vi "SendCTREPCMProtocol.vi"(7 "Send":bool, 9 "Initialize":bool, 10 "Previous":T1={"type"="CTREPCM", "device"="", "name"="", "data"={"<init"=FALSE, ">on"=FALSE, "<closed_loop"=FALSE, ">pressure_switch"=FALSE, ">current"=0.0}}, 11 "Current":T1={"type"="CTREPCM", "device"="", "name"="", "data"={"<init"=FALSE, ">on"=FALSE, "<closed_loop"=FALSE, ">pressure_switch"=FALSE, ">current"=0.0}}) -> ()   [LabVIEW 2019]
uses:
  CTREPCM Data proto.ctl
  CTREPCM proto.ctl
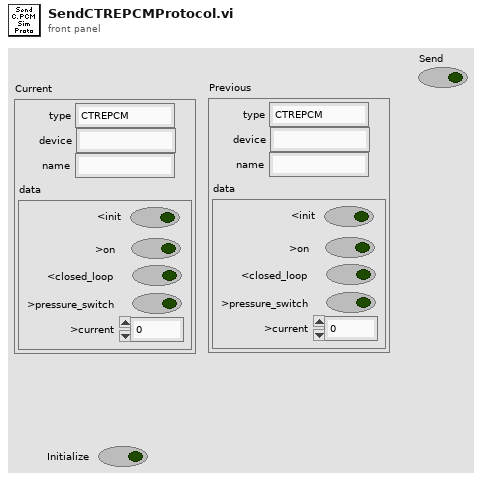
[diagram p1: front panel]
types:
  T1 = typedef "CTREPCM proto.ctl" = cluster{"type":string, "device":string, "name":string, "data":T2}
  T2 = typedef "CTREPCM Data proto.ctl" = cluster{"<init":bool, ">on":bool, "<closed_loop":bool, ">pressure_switch":bool, ">current":dbl}
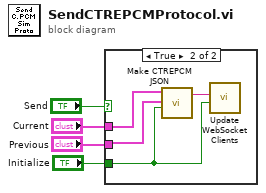
[diagram p0: block diagram]
diagram:
  n1 = case shown="True" "Send" {
    tunnel: "Current" -> [_ w8]
    tunnel: "Previous" -> [_ w7]
    tunnel: "Initialize" -> [_ w6]
    frame False {
    }
    frame True {
      n2 = call "Make CTREPCM JSON.vi"("Force"=w6, "Previous"=w7, "New"=w8) -> ("delta JSON"=w5:string)  [unwired: 8 in]
      n3 = call "Update WebSocket Clients.vi"("Initialize"=w6, "delta JSON"=w5) -> ()  [unwired: 10 in]
    }
  }
